vi "Read State.vi"(11 "Pump_1AI_1DO_2DI in":refnum<class "ValveModbus.lvclass">) -> (2 "StateValveModbus":T1=enum."OPEN")   [LabVIEW 2019, in "ValveModbus.lvclass"]
uses:
  ValveModbus.lvclass
  TypeDef/StateValveModbus.ctl
  ValveModbus.lvclass/ValveModbus.ctl
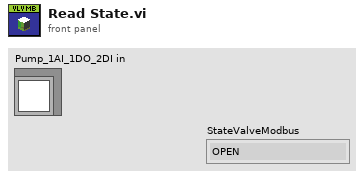
[diagram p1: front panel]
types:
  T1 = typedef "StateValveModbus.ctl" = enum16{"IDLE", "OPEN", "CLOSE", "OPENING", "CLOSING", "STOP"}
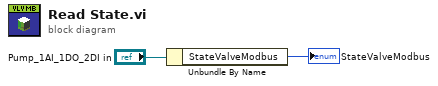
[diagram p0: block diagram]
diagram:
  n1 = Unbundle By Name("Pump_1AI_1DO_2DI in") -> ("StateValveModbus"=→"StateValveModbus":T1)
